vi "Nested Status.vi"(11 "jettl Queue Actor in":refnum<class "jettl Queue Actor.lvclass">) -> (0 "Nested Count":i32, 1 "Nested Aliases":string[](array[string]), 2 "Any Exist?":bool)   [LabVIEW 2021, in "jettl.lvlib" / "jettl Queue Actor.lvlib" / "jettl Queue Actor.lvclass"]
uses:
  jettl Queue Actor.lvclass
  jettl Queue Actor.lvclass/jettl Queue Actor.ctl
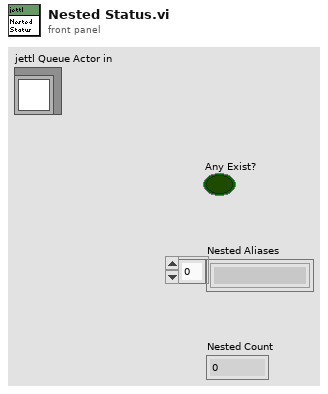
[diagram p1: front panel]
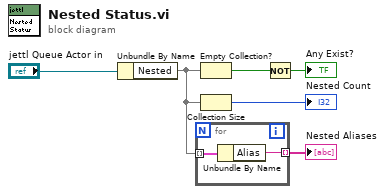
[diagram p0: block diagram]
diagram:
  n1 = Unbundle By Name("jettl Queue Actor in") -> ("Nested"=w3:map{string, refnum<data-value>})
  n2 = for {
    tunnel: [w7] -> w5 mode=indexing
    tunnel: w3 -> [w8] mode=indexing
    n3 = Unbundle By Name(w8) -> ("Alias"=w7:string)
  }
  "Nested Aliases" <- w5
  n4 = Empty Collection?(1:w3) -> (0:w2:bool)
  n5 = Collection Size(1:w3) -> (0:→"Nested Count":i32)
  n6 = Not(x=w2) -> (.not. x?=→"Any Exist?":bool)
